vi "ReadServerErrorStatus.vi"(8 "error in":errorcluster) -> (3 "Error Status":string="1")   [LabVIEW 2011]
uses:
  Typedefs/ServerErrorFilePath.ctl
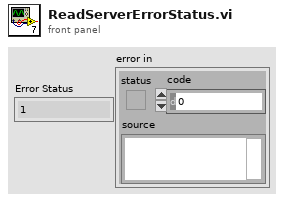
[diagram p1: front panel]
types:
  T1 = enum16{"open", "replace", "create", "open or create", "replace or create", "replace or create with confirmation"}
  T2 = typedef "ServerErrorFilePath.ctl" = path
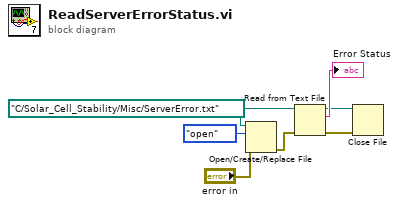
[diagram p0: block diagram]
diagram:
  w5 = T2 path "C:/Solar_Cell_Stability/Misc/ServerError.txt" ("file path (use dialog)")
  n1 = Open/Create/Replace File(file path (use dialog)=w5, error in="error in", operation (0:open)=T1."open") -> (error out=w4:errorcluster)  [unwired: 3 in, 2 out]
  n2 = Read from Text File(file (use dialog)=w5, error in=w4) -> (refnum out=w2:refnum<file>, text=→"Error Status":string, error out=w3:errorcluster)  [unwired: 2 in, 1 out]
  n3 = Close File(refnum=w2, error in=w3) -> ()  [unwired: 2 out]
